vi "Vision Sub.vi"(9 "Gyro Angle":dbl, 11 "X? Input":dbl) -> (1 "Right Motors":dbl, 2 "Left Motors":dbl, 3 "Nothing In Sight":bool)   [LabVIEW 2016]
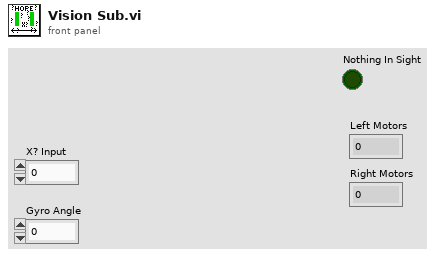
[diagram p1: front panel]
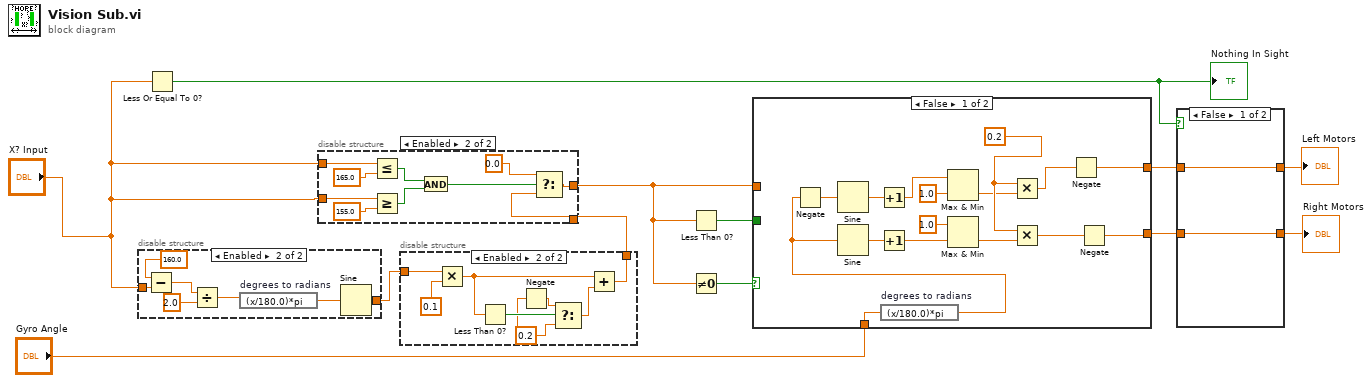
[diagram p0: block diagram]
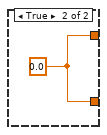
[diagram p2: hidden frame]
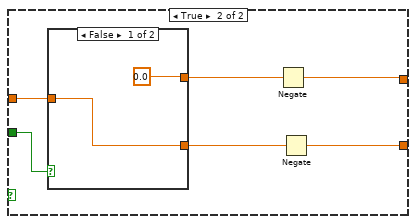
[diagram p6: hidden frame]
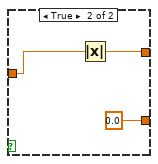
[diagram p7: hidden frame]
diagram:
  n1 = disable-structure shown="Enabled" {
    disable-tunnel: "X? Input" -> [_ w14]
    disable-tunnel: [_ w13] -> w7
    frame Disabled {
    }
    frame Enabled {
      n2 = Subtract(x=160.0, y=w14) -> (x-y=w16:dbl)
      n3 = Divide(x=w16, y=2.0) -> (x/y=w18:dbl)
      n4 = expression code="(x/180.0)*pi" "degrees to radians"(w18) -> (w19:dbl)
      n5 = Sine(x=w19) -> (sin(x)=w13:dbl)
    }
  }
  n6 = Less Or Equal To 0?(x="X? Input") -> (x <= 0?=w5:bool)
  "Nothing In Sight" <- w5
  n7 = disable-structure shown="Enabled" {
    disable-tunnel: w7 -> [_ w22]
    disable-tunnel: [_ w21] -> w6
    frame Disabled {
    }
    frame Enabled {
      w20 = 0.2 ("f")
      n8 = Multiply(x=w22, y=0.1) -> (x*y=w26:dbl)
      n9 = Less Than 0?(x=w26) -> (x < 0?=w24:bool)
      n10 = Negate(x=w20) -> (-x=w27:dbl)
      n11 = Select(t=w27, s=w24, f=w20) -> (s? t:f=w25:dbl)
      n12 = Add(x=w26, y=w25) -> (x+y=w21:dbl)
    }
  }
  n13 = disable-structure shown="Enabled" {
    disable-tunnel: [_ w31] -> w11
    disable-tunnel: w6 -> [_ w30]
    disable-tunnel: "X? Input" -> [_ w29]
    disable-tunnel: "X? Input" -> [_ w28]
    frame Disabled {
    }
    frame Enabled {
      n14 = Less Or Equal?(x=w29, y=165.0) -> (x <= y?=w35:bool)
      n15 = Greater Or Equal?(x=w28, y=155.0) -> (x >= y?=w34:bool)
      n16 = And(x=w35, y=w34) -> (x .and. y?=w37:bool)
      n17 = Select(t=0.0, s=w37, f=w30) -> (s? t:f=w31:dbl)
    }
  }
  n18 = Less Than 0?(x=w11) -> (x < 0?=w12:bool)
  n19 = Not Equal To 0?(x=w11) -> (x != 0?=w10:bool)
  n20 = case shown="False" w10 {
    tunnel: w12 -> [_ w59]
    tunnel: w11 -> [_ w58]
    tunnel: [w39 w54] -> w8
    tunnel: [w40 w55] -> w9
    tunnel: "Gyro Angle" -> [w38 _]
    frame False {
      w53 = 0.2 ("x")
      n21 = expression code="(x/180.0)*pi" "degrees to radians"(w38) -> (w52:dbl)
      n22 = Negate(x=w52) -> (-x=w47:dbl)
      n23 = Sine(x=w47) -> (sin(x)=w45:dbl)
      n24 = Sine(x=w52) -> (sin(x)=w43:dbl)
      n25 = Increment(x=w45) -> (x+1=w46:dbl)
      n26 = Increment(x=w43) -> (x+1=w44:dbl)
      n27 = Max & Min(x=w46, y=1.0) -> (min(x,y)=w49:dbl)  [unwired: 1 out]
      n28 = Max & Min(x=1.0, y=w44) -> (min(x,y)=w48:dbl)  [unwired: 1 out]
      n29 = Multiply(x=w53, y=w49) -> (x*y=w50:dbl)
      n30 = Multiply(x=w53, y=w48) -> (x*y=w51:dbl)
      n31 = Negate(x=w50) -> (-x=w40:dbl)
      n32 = Negate(x=w51) -> (-x=w39:dbl)
    }
    frame True {
      n33 = case shown="False" w59 {
        tunnel: w58 -> [w60 w64]
        tunnel: [w60 0.0] -> w57
        tunnel: [0.0 w63] -> w56
        frame False {
        }
        frame True {
          n34 = Absolute Value(x=w64) -> (abs(x)=w63:dbl)
        }
      }
      n35 = Negate(x=w56) -> (-x=w55:dbl)
      n36 = Negate(x=w57) -> (-x=w54:dbl)
    }
  }
  n37 = case shown="False" w5 {
    tunnel: w9 -> [w66 _]
    tunnel: w8 -> [w65 _]
    tunnel: [w65 w67] -> w4
    tunnel: [w66 w67] -> w3
    frame False {
    }
    frame True {
      w67 = 0.0
    }
  }
  "Left Motors" <- w3
  "Right Motors" <- w4
